vi "DependencyViewer_OnCommand.vi"(10 "Command Tag":string, 11 "Object":u64) -> ()   [LabVIEW 2020]
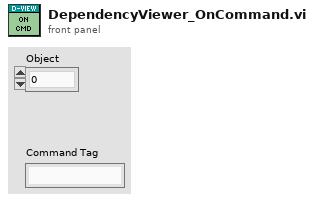
[diagram p1: front panel]
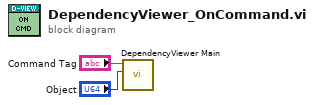
[diagram p0: block diagram]
diagram:
  n1 = call "DependencyViewer Main.vi"("Object"="Object", "Sub Command"="Command Tag") -> ()  [unwired: 10 in]
